vi "OnUpdate.vi"(8 "error in (no error)":errorcluster) -> (0 "error out":errorcluster)   [LabVIEW 2020, in "WebServiceImporter.lvlib" / "Main Panel.lvlib" / "Finish.lvlib"]
uses:
  <vilib>/Platform/WebService/Main Panel/Pages/Finish/Finish.lvlib
  <vilib>/Platform/WebService/Main Panel/Pages/Finish/Events/Events.lvlib
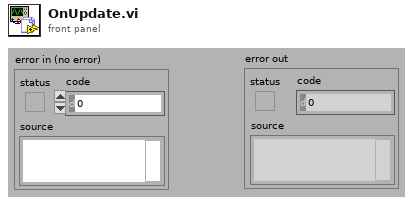
[diagram p1: front panel]
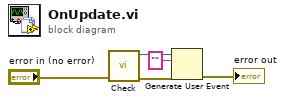
[diagram p0: block diagram]
diagram:
  n1 = call <vilib>:"Check.vi"("error in (no error)"="error in (no error)") -> ("error out"=w3:errorcluster, "user event (out)"=w4:refnum<user-event>)  [unwired: 9 in]
  n2 = Generate User Event(user event=w4, event data cluster="" ("event data"), error in=w3) -> (error out=→"error out":errorcluster)  [unwired: 1 in, 1 out]
